vi "simulated bridge.vi"(2 "s4":bool, 3 "s3":bool, 4 "s2":bool, 5 "s1":bool) -> (0 "Free Wheel":bool, 1 "Motor voltage":i8)   [LabVIEW 2017]
panel:
  out "Left":bool
  out "Right":bool
  out "Brake":bool
  out "Short":bool
  out "Q4":bool
  out "Q2":bool
  out "Q3":bool
  out "Q1":bool
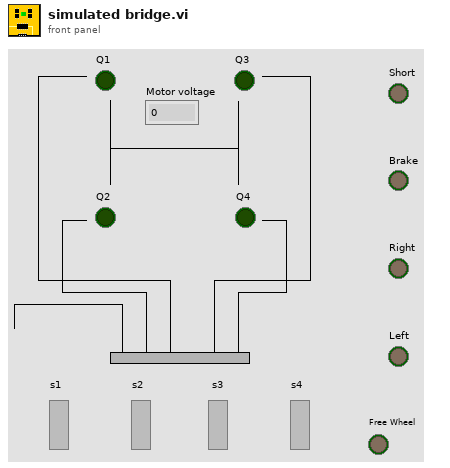
[diagram p1: front panel]
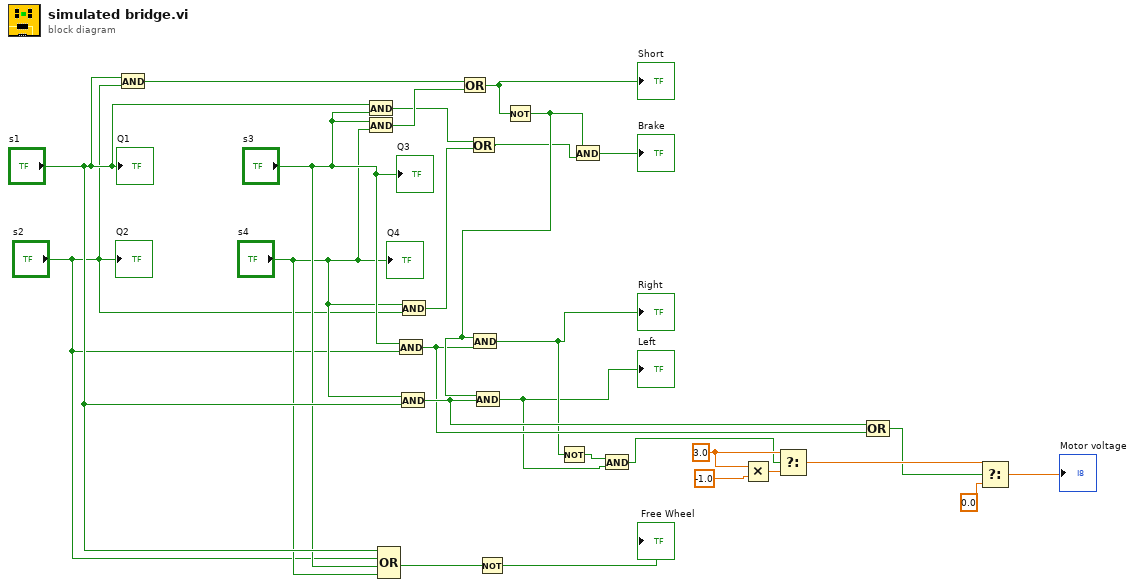
[diagram p0: block diagram]
diagram:
  w16 = 3.0 ("t")
  n1 = And(x="s1", y="s2") -> (x .and. y?=w27:bool)
  n2 = And(x="s1", y="s3") -> (x .and. y?=w23:bool)
  n3 = And(x="s3", y="s4") -> (x .and. y?=w26:bool)
  n4 = Compound Arithmetic op=OR("s1", "s2", "s3", "s4") -> (w12:bool)
  n5 = And(x="s3", y="s2") -> (x .and. y?=w9:bool)
  n6 = And(x="s4", y="s1") -> (x .and. y?=w10:bool)
  n7 = And(x="s4", y="s2") -> (x .and. y?=w22:bool)
  n8 = Or(x=w27, y=w26) -> (x .or. y?=w3:bool)
  "Short" <- w3
  n9 = Or(x=w23, y=w22) -> (x .or. y?=w24:bool)
  n10 = Not(x=w12) -> (.not. x?=→"Free Wheel":bool)
  n11 = Not(x=w3) -> (.not. x?=w25:bool)
  n12 = And(x=w25, y=w9) -> (x .and. y?=w6:bool)
  "Right" <- w6
  n13 = And(x=w25, y=w10) -> (x .and. y?=w5:bool)
  "Left" <- w5
  n14 = Not(x=w6) -> (.not. x?=w7:bool)
  n15 = And(x=w25, y=w24) -> (x .and. y?=→"Brake":bool)
  n16 = And(x=w7, y=w5) -> (x .and. y?=w4:bool)
  n17 = Multiply(x=w16, y=-1.0) -> (x*y=w14:dbl)
  n18 = Select(t=w16, s=w4, f=w14) -> (s? t:f=w17:dbl)
  n19 = Compound Arithmetic op=OR(w10, w9) -> (w8:bool)
  n20 = Select(t=w17, s=w8, f=0.0) -> (s? t:f=→"Motor voltage":dbl)
  "Q1" <- "s1"
  "Q3" <- "s3"
  "Q2" <- "s2"
  "Q4" <- "s4"
